vi "zjistiPruchodyNulou.vi"(8 "smerPruchodu":bool, 10 "prahDetekce":dbl, 11 "vstupniSignal":waveform(dbl)) -> (3 "vsechnyPruchody":i32[](array[numeric]))   [LabVIEW 2018]
panel:
  # "Vstupy:"
  # "Výstupy:"
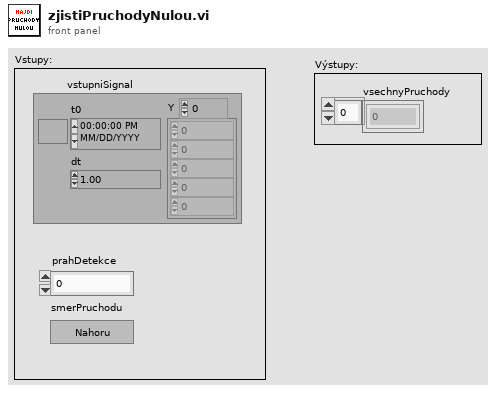
[diagram p1: front panel]
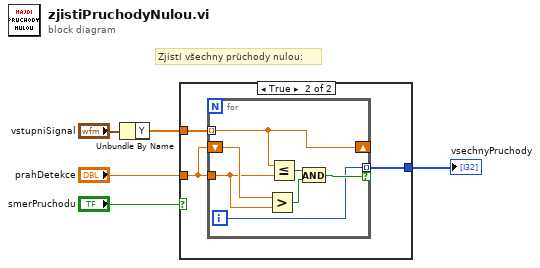
[diagram p0: block diagram]
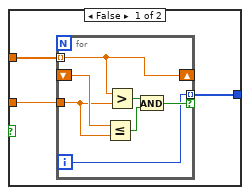
[diagram p2: hidden frame]
diagram:
  # "Zjistí všechny prùchody nulou:"
  n1 = Unbundle By Name("vstupniSignal") -> ("Y"=w1:dbl[])
  n2 = case shown="True" "smerPruchodu" {
    tunnel: [w6 w18] -> w4
    tunnel: w1 -> [w8 w17]
    tunnel: "prahDetekce" -> [w7 w16]
    frame False {
      n3 = for {
        tunnel: w8 -> [w15] mode=indexing
        shift-right: [w15] -> _
        shift-left: _ -> [w14]
        tunnel: w7 -> [w13]
        tunnel: [w9] -> w6 mode=indexing if=w10
        i -> [w9]
        n4 = Less Or Equal?(x=w14, y=w13) -> (x <= y?=w11:bool)
        n5 = Greater?(x=w15, y=w13) -> (0:w12:bool)
        n6 = And(x=w12, y=w11) -> (x .and. y?=w10:bool)
      }
    }
    frame True {
      n7 = for {
        tunnel: w17 -> [w25] mode=indexing
        shift-right: [w25] -> _
        shift-left: w16 -> [w24]
        tunnel: w16 -> [w23]
        tunnel: [w19] -> w18 mode=indexing if=w20
        i -> [w19]
        n8 = Greater?(x=w24, y=w23) -> (0:w21:bool)
        n9 = Less Or Equal?(x=w25, y=w23) -> (x <= y?=w22:bool)
        n10 = And(x=w22, y=w21) -> (x .and. y?=w20:bool)
      }
    }
  }
  "vsechnyPruchody" <- w4
